vi "Create_pos_for_all_ch.vi"() -> (1 "Positions for all Ch":T1(array[cluster]) {"Z" format="%.2f"; "Y" format="%.2f"; "X" format="%.2f"})   [LabVIEW 2010]
uses:
  Globals/Meas_global.vi
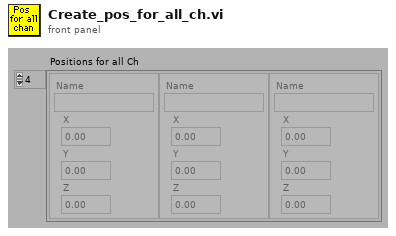
[diagram p1: front panel]
types:
  T1 = cluster{"Name":string, "X":dbl, "Y":dbl, "Z":dbl}[]
  T2 = typedef "Analysis_info_cluster.ctl" = cluster{"Colour":u32, "Inst type":T3, "Inst name":string, "Symbol":string, "Code name":string, "Extra Info":string, "Inst Array":T4, "Index":i32, "Voltage Index":i32, "Extra Titles":string[], "Extra Values":string[]}
  T3 = typedef "Inst_type.ctl" = enum16{"Propeller anemometer", "Raw voltage", "Pressure Transducer", "Pitot-static tube", "Preston tube", "Hot wire", "Cross wire 1", "Cross wire 2", "Generic Linear", "Generic Polynomial", "Generic BackPoly", "Fast FID", "Thermocouple", "Cold wire", "Pulsed Wire", "LDA Vel", "LDA Tran time", "LDA Arr time"}
  T4 = typedef "Instrument_Array.ctl" = enum16{"PWA", "LDA", "Analogue"}
  T5 = cluster{"Name":string, "X":dbl, "Y":dbl, "Z":dbl}
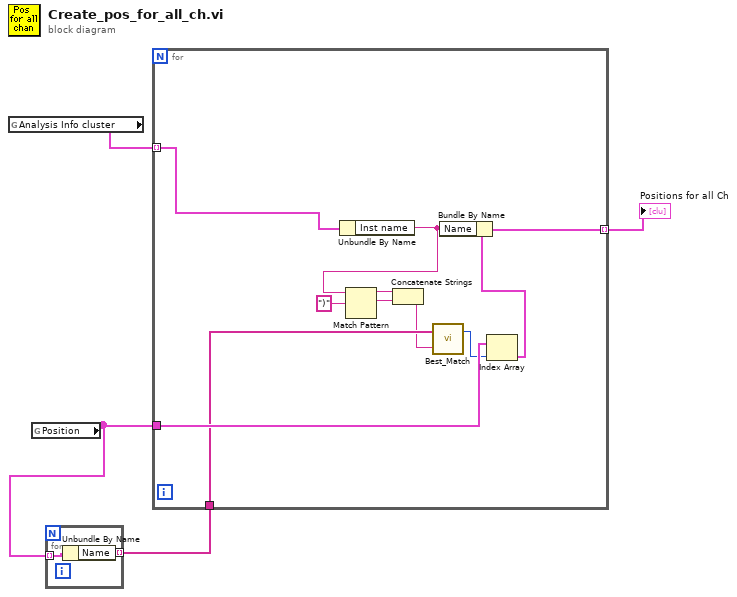
[diagram p0: block diagram]
diagram:
  n1 = global read "Meas_global.vi" "Analysis Info cluster"() -> (w4:T2[])
  n2 = global read "Meas_global.vi" "Position"() -> (w3:T1)
  n3 = for {
    tunnel: w3 -> [w6] mode=indexing
    tunnel: [w5] -> w2 mode=indexing
    n4 = Unbundle By Name(w6) -> ("Name"=w5:string)
  }
  n5 = for {
    tunnel: w3 -> [w17]
    tunnel: w4 -> [w11] mode=indexing
    tunnel: w2 -> [w9]
    tunnel: [w10] -> w1 mode=indexing
    n6 = Unbundle By Name(w11) -> ("Inst name"=w16:string)
    n7 = Match Pattern(string=w16, regular expression=")") -> (before substring=w14:string, match substring=w13:string)  [unwired: 1 in, 2 out]
    n8 = Concatenate Strings(w14, w13) -> (w8:string)
    n9 = call "Best_Match.vi"("Input String"=w8, "String Options"=w9) -> ("index of element"=w7:i32)  [unwired: 1 out]
    n10 = Index Array(array=w17, index=w7) -> (element=w12:T5)
    n11 = Bundle By Name(cluster=w12, "Name"=w16) -> (w10:T5)
  }
  "Positions for all Ch" <- w1
